vi "Post-Build Action.vi"(5 "Files Generated by Build":path[](array[path]), 6 "Top Level/Always Included VIs":path[](array[path]), 7 "Destination Path":path, 8 "error in (no error)":errorcluster, 9 "Target Name":string, 10 "Build Specification Name":string, 11 "Project Path":path) -> (0 "error out":errorcluster)   [LabVIEW 2021, in "AC_Audio ADC.lvlib"]
uses:
  AC_Audio ADC.lvlib
  MeasurementPlugin.lvclass
  C:/Program Files/National Instruments/LabVIEW 2021/vi.lib/MeasurementLink/MeasurementLink Measurement Server/Classes/MeasurementPluginService/MeasurementPluginService.lvclass
  shared/audio adc shared.lvlib
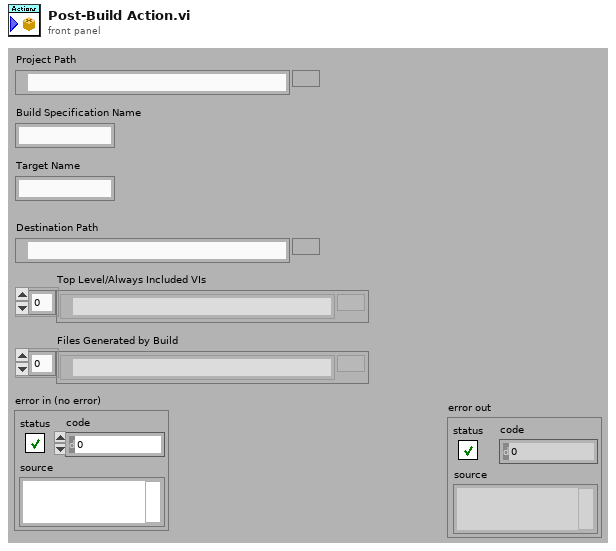
[diagram p1: front panel]
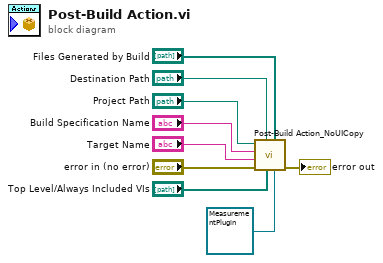
[diagram p0: block diagram]
diagram:
  n1 = call "Post-Build Action_NoUICopy.vi"("Measurement"=refnum<class "MeasurementPlugin.lvclass"> refnum ("MeasurementLink Measurement Template.lvlib:MeasurementPlugin.lvclass"), "Files Generated by Build"="Files Generated by Build", "Top Level/Always Included VIs"="Top Level/Always Included VIs", "Destination Path"="Destination Path", "error in (no error)"="error in (no error)", "Target Name"="Target Name", "Build Specification Name"="Build Specification Name", "Project Path"="Project Path") -> ("error out"=→"error out":errorcluster)  [unwired: 3 in]
